vi "Erease Data(Clear Data).vi"(6 "Variant in":variant, 7 "Shift Pressed?":bool, 8 "error in (no error)":errorcluster, 10 "QD Combo Box Ref":refnum<vi>, 11 "QD Launch VI Ref":refnum<vi>) -> (0 "error out":errorcluster, 4 "Variant out":variant)   [LabVIEW 2015, in "QD_Erease Data.lvlib"]
doc: "Clear control/Constant's data. Supported type:\n- Array\n- String\n- Listbox\n- MulticolumnListBox\n- Numeric\n- Table\n- Tree\n\nDefault Shortcut - [E]"
uses:
  QD_Erease Data.lvlib
panel:
  # "Do not change the connector pane of this VI.\n\nSee the block diagram for directions on how to use this template."
  # "Specify the name of the Undo transaction"
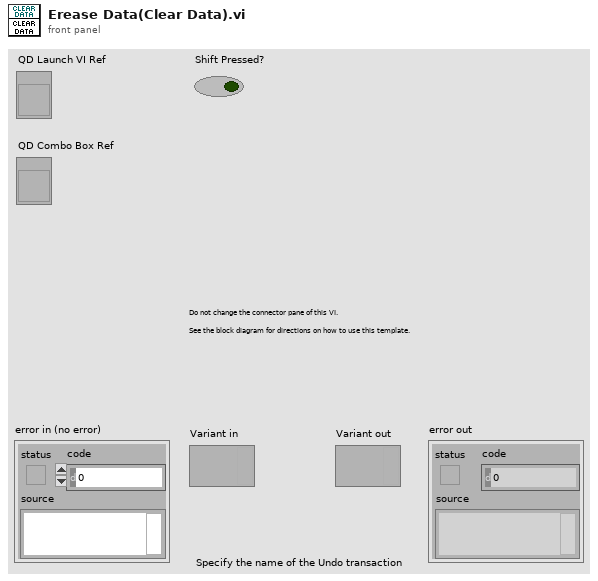
[diagram p1: front panel]
types:
  T1 = typedef "Type Descriptor Enumeration__ogtk.ctl" = enum8{"<Null>", "I8", "I16", "I32", "I64", "U8", "U16", "U32", "U64", "SGL", "DBL", "EXT", "CSG", "CDB", "CXT", "0x0F", "0x10", "0x11", "0x12", "0x13", "0x14", "Enum U8", "Enum U16", "Enum U32", "Enum U64", "SGL PQ", "DBL PQ", "EXT PQ", "CSG PQ", "CDB PQ", "CXT PQ", "0x1F", "0x20", "Boolean", "0x22", "0x23", "0x24", "0x25", "0x26", "0x27", "0x28", "0x29", "0x2A", "0x2B", "0x2C", "0x2D", "0x2E", "0x2F", "String", "0x31", "Path", "Pict", "0x34", "0x35", "0x36", "DAQ", "0x38", "0x39", "0x3A", "0x3B", "0x3C", "0x3D", "0x3E", "0x3F", "Array", "0x41", "0x42", "0x43", "0x44", "0x45", "0x46", "0x47", "0x48", "0x49", "0x4A", "0x4B", "0x4C", "0x4D", "0x4E", "0x4F", "Cluster", "0x51", "0x52", "Variant", "Waveform", "0x55", "0x56", "0x57", "0x58", "0x59", "0x5A", "0x5B", "0x5C", "0x5D", "0x5E", "Fixed Point", "0x60", "0x61", "0x62", "0x63", "0x64", "0x65", "0x66", "0x67", "0x68", "0x69", "0x6A", "0x6B", "0x6C", "0x6D", "0x6E", "0x6F", "Refnum", "0x71", "0x72", "Set Collection", "Map Collection"}
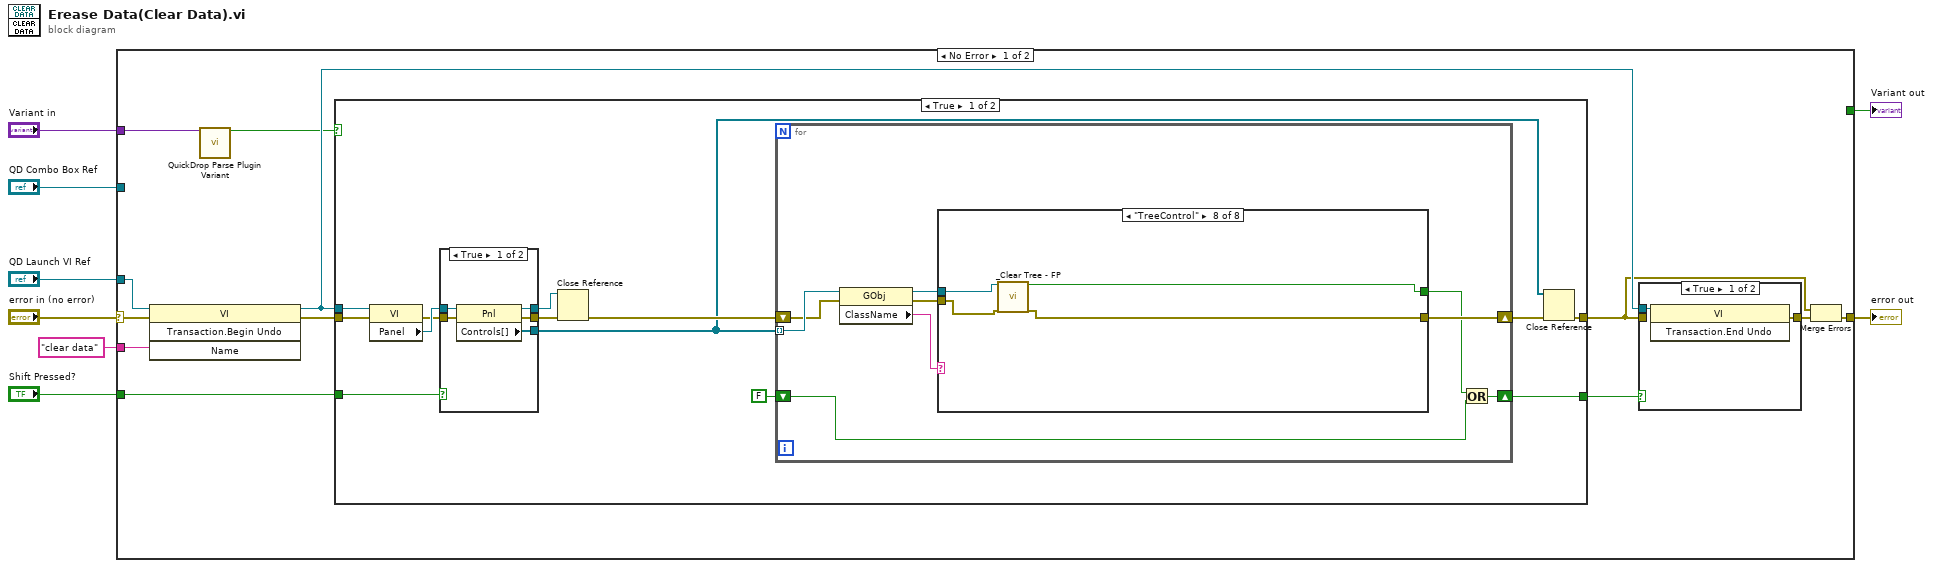
[diagram p0: block diagram]
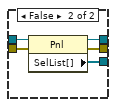
[diagram p2: hidden frame]
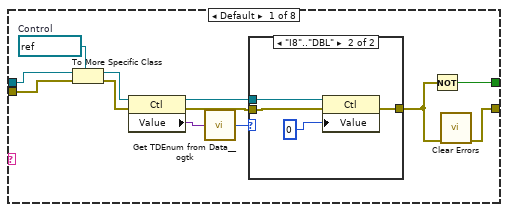
[diagram p3: hidden frame]
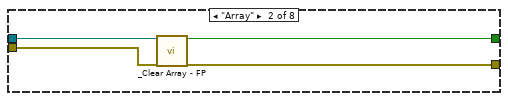
[diagram p5: hidden frame]
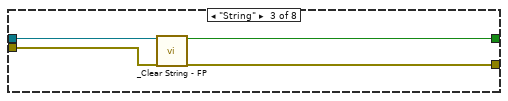
[diagram p6: hidden frame]
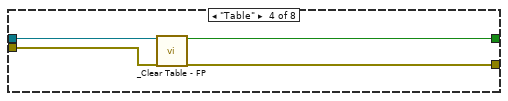
[diagram p7: hidden frame]
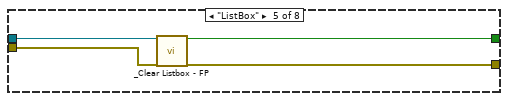
[diagram p8: hidden frame]
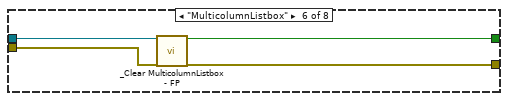
[diagram p9: hidden frame]
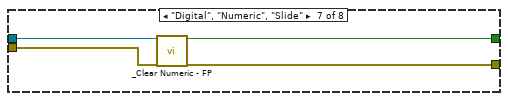
[diagram p10: hidden frame]
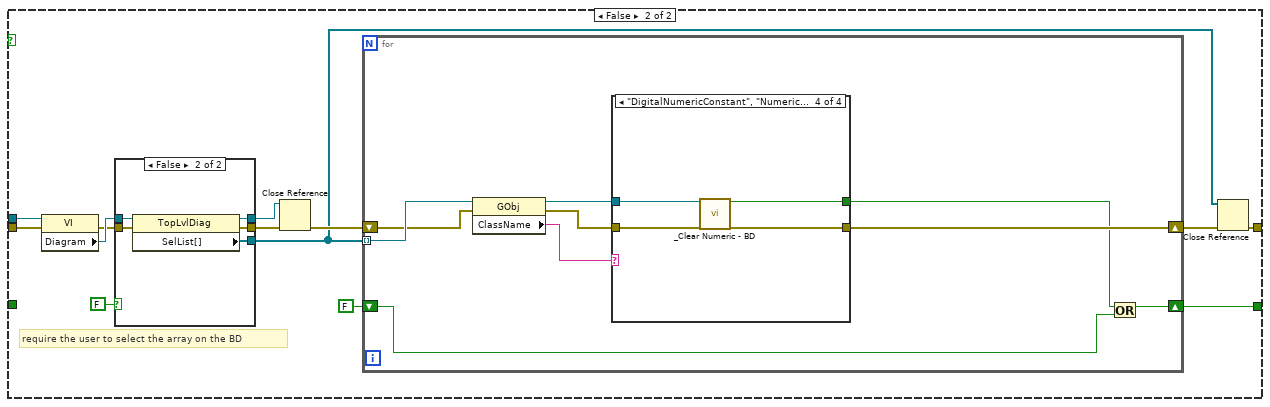
[diagram p11: hidden frame]
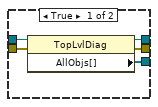
[diagram p12: hidden frame]
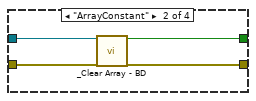
[diagram p14: hidden frame]
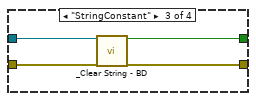
[diagram p15: hidden frame]
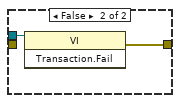
[diagram p16: hidden frame]
diagram:
  n1 = case shown="No Error" "error in (no error)" {
    selector: "error in (no error)" -> [w20 w148]
    tunnel: [w10 w148] -> w7
    tunnel: "QD Launch VI Ref" -> [w19 _]
    tunnel: "Shift Pressed?" -> [w14 _]
    tunnel: "QD Combo Box Ref" -> [_ _]
    tunnel: "Variant in" -> [w21 _]
    tunnel: "clear data" ("Undo Name") -> [w18 _]
    tunnel: [TRUE _] -> w1
    frame No Error {
      n2 = invoke class="VI" method="Transaction.Begin Undo"(reference=w19, error in=w20, "Name"=w18) -> (reference out=w13:refnum<vi>, error out=w16:errorcluster)  [unwired: 1 in, 2 out]
      n3 = call <vilib>:"QuickDrop Parse Plugin Variant.vi"("QDKS Variant in"=w21) -> ("QD Launch VI Panel?"=w12:bool)  [unwired: 12 in, 2 out]
      n4 = case shown="True" w12 {
        tunnel: w16 -> [w34 w111]
        tunnel: [w30 w107] -> w9
        tunnel: w14 -> [w25 _]
        tunnel: w13 -> [w28 w105]
        tunnel: [w23 w101] -> w11
        frame True {
          n5 = property class="VI"(reference=w28, error in=w34) -> (error out=w26:errorcluster, "Panel"=w27:refnum<vi>)  [unwired: 1 out]
          n6 = case shown="True" w25 {
            tunnel: [w39 w44] -> w32
            tunnel: [w38 w43] -> w31
            tunnel: [w37 w42] -> w29
            tunnel: w27 -> [w36 w41]
            tunnel: w26 -> [w35 w40]
            frame True {
              n7 = property class="Pnl"(reference=w36, error in=w35) -> (reference out=w38:refnum<vi>, error out=w39:errorcluster, "Controls[]"=w37:refnum<vi>[])
            }
            frame False {
              n8 = property class="Pnl"(reference=w41, error in=w40) -> (reference out=w43:refnum<vi>, error out=w44:errorcluster, "SelList[]"=w42:refnum<vi>[])
            }
          }
          n9 = Close Reference(reference=w31, error in (no error)=w32) -> (error out=w33:errorcluster)
          n10 = for {
            shift-right: [w53] -> w24
            shift-left: w33 -> [w47]
            tunnel: w29 -> [w52] mode=indexing
            shift-right: [w50] -> w23
            shift-left: FALSE -> [w49]
            n11 = property class="GObj"(reference=w52, error in=w47) -> (reference out=w48:refnum<vi>, error out=w46:errorcluster, "ClassName"=w45:string)
            n12 = case shown="\"TreeControl\"" w45 {
              tunnel: [w54 w74 w78 w82 w86 w90 w94 w96] -> w53
              tunnel: [w55 w73 w77 w81 w85 w89 w93 w95] -> w51
              tunnel: w48 -> [w64 w72 w76 w80 w84 w88 w92 w98]
              tunnel: w46 -> [w63 w71 w75 w79 w83 w87 w91 w97]
              frame Default {
                w65 = refnum<vi> refnum  # Control
                n13 = To More Specific Class(target class=w65, reference=w64, error in=w63) -> (specific class reference=w62:refnum<vi>, error out=w61:errorcluster)
                n14 = property class="Ctl"(reference=w62, error in=w61) -> (reference out=w58:refnum<vi>, error out=w57:errorcluster, "Value"=w60:variant)
                n15 = call <userlib>:"Get TDEnum from Data__ogtk.vi"("Data"=w60) -> ("Type Descriptor Enumeration"=w59:T1)  [unwired: 4 in]
                n16 = case shown="\"I8\"..\"DBL\"" w59 {
                  tunnel: w58 -> [_ w70]
                  tunnel: w57 -> [w66 w69]
                  tunnel: [w66 w68] -> w56
                  frame "<Null>", Default {
                  }
                  frame "I8".."DBL" {
                    n17 = property class="Ctl"(reference=w70, error in=w69, "Value"=0) -> (error out=w68:errorcluster)  [unwired: 1 out]
                  }
                }
                n18 = Not(x=w56) -> (.not. x?=w55:bool)
                n19 = call <vilib>:"Clear Errors.vi"("error in (no error)"=w56) -> ("error out"=w54:errorcluster)  [unwired: 5 in, 1 out]
              }
              frame "Array" {
                n20 = call "_Clear Array - FP.vi"("GObject in"=w72, "error in (no error)"=w71) -> ("changed?"=w73:bool, "error out"=w74:errorcluster)  [unwired: 16 in]
              }
              frame "String" {
                n21 = call "_Clear String - FP.vi"("GObject in"=w76, "error in (no error)"=w75) -> ("changed?"=w77:bool, "error out"=w78:errorcluster)  [unwired: 16 in]
              }
              frame "Table" {
                n22 = call "_Clear Table - FP.vi"("GObject in"=w80, "error in (no error)"=w79) -> ("changed?"=w81:bool, "error out"=w82:errorcluster)  [unwired: 16 in]
              }
              frame "ListBox" {
                n23 = call "_Clear Listbox - FP.vi"("GObject in"=w84, "error in (no error)"=w83) -> ("changed?"=w85:bool, "error out"=w86:errorcluster)  [unwired: 16 in]
              }
              frame "MulticolumnListbox" {
                n24 = call "_Clear MulticolumnListbox - FP.vi"("GObject in"=w88, "error in (no error)"=w87) -> ("changed?"=w89:bool, "error out"=w90:errorcluster)  [unwired: 16 in]
              }
              frame "Digital", "Numeric", "Slide" {
                n25 = call "_Clear Numeric - FP.vi"("GObject in"=w92, "error in (no error)"=w91) -> ("changed?"=w93:bool, "error out"=w94:errorcluster)  [unwired: 16 in]
              }
              frame "TreeControl" {
                n26 = call "_Clear Tree - FP.vi"("GObject in"=w98, "error in (no error)"=w97) -> ("changed?"=w95:bool, "error out"=w96:errorcluster)  [unwired: 16 in]
              }
            }
            n27 = Or(x=w51, y=w49) -> (x .or. y?=w50:bool)
          }
          n28 = Close Reference(reference=w29, error in (no error)=w24) -> (error out=w30:errorcluster)
        }
        frame False {
          # "require the user to select the array on the BD"
          n29 = property class="VI"(reference=w105, error in=w111) -> (error out=w103:errorcluster, "Diagram"=w104:refnum<vi>)  [unwired: 1 out]
          n30 = case shown="False" FALSE {
            tunnel: [w116 w121] -> w109
            tunnel: [w115 w120] -> w108
            tunnel: [w114 w119] -> w106
            tunnel: w104 -> [w113 w118]
            tunnel: w103 -> [w112 w117]
            frame True {
              n31 = property class="TopLvlDiag"(reference=w113, error in=w112) -> (reference out=w115:refnum<vi>, error out=w116:errorcluster, "AllObjs[]"=w114:refnum<vi>[])
            }
            frame False {
              n32 = property class="TopLvlDiag"(reference=w118, error in=w117) -> (reference out=w120:refnum<vi>, error out=w121:errorcluster, "SelList[]"=w119:refnum<vi>[])
            }
          }
          n33 = Close Reference(reference=w108, error in (no error)=w109) -> (error out=w110:errorcluster)
          n34 = for {
            shift-right: [w130] -> w102
            shift-left: w110 -> [w124]
            tunnel: w106 -> [w129] mode=indexing
            shift-right: [w127] -> w101
            shift-left: FALSE -> [w126]
            n35 = property class="GObj"(reference=w129, error in=w124) -> (reference out=w125:refnum<vi>, error out=w123:errorcluster, "ClassName"=w122:string)
            n36 = case shown="\"DigitalNumericConstant\", \"NumericConstant\"" w122 {
              tunnel: [w131 w135 w139 w143] -> w130
              tunnel: [_ w134 w138 w142] -> w128
              tunnel: w125 -> [_ w133 w137 w141]
              tunnel: w123 -> [w131 w132 w136 w140]
              frame Default {
              }
              frame "ArrayConstant" {
                n37 = call "_Clear Array - BD.vi"("GObject in"=w133, "error in (no error)"=w132) -> ("changed?"=w134:bool, "error out"=w135:errorcluster)  [unwired: 16 in]
              }
              frame "StringConstant" {
                n38 = call "_Clear String - BD.vi"("GObject in"=w137, "error in (no error)"=w136) -> ("changed?"=w138:bool, "error out"=w139:errorcluster)  [unwired: 16 in]
              }
              frame "DigitalNumericConstant", "NumericConstant" {
                n39 = call "_Clear Numeric - BD.vi"("GObject in"=w141, "error in (no error)"=w140) -> ("changed?"=w142:bool, "error out"=w143:errorcluster)  [unwired: 16 in]
              }
            }
            n40 = Or(x=w128, y=w126) -> (x .or. y?=w127:bool)
          }
          n41 = Close Reference(reference=w106, error in (no error)=w102) -> (error out=w107:errorcluster)
        }
      }
      n42 = case shown="True" w11 {
        tunnel: w13 -> [w144 w146]
        tunnel: [w145 w147] -> w15
        tunnel: w9 -> [_ _]
        frame True {
          n43 = invoke class="VI" method="Transaction.End Undo"(reference=w144) -> (error out=w145:errorcluster)  [unwired: 2 in, 2 out]
        }
        frame False {
          n44 = invoke class="VI" method="Transaction.Fail"(reference=w146) -> (error out=w147:errorcluster)  [unwired: 2 in, 2 out]
        }
      }
      n45 = Merge Errors(w9, w15) -> (w10:errorcluster)
    }
    frame Error {
    }
  }
  "error out" <- w7
  "Variant out" <- w1
